vi "XML ( Open ).vi"(8 "error in (no error)":errorcluster, 10 "XML document":path caption="path to XML document", 11 "XML in":refnum<class "XML.lvclass">) -> (0 "error out":errorcluster, 3 "XML out":refnum<class "XML.lvclass">)   [LabVIEW 2018, in "XML.lvlib" / "XML.lvclass"]
uses:
  XML.lvclass
  XML.lvclass/XML.ctl
  <vilib>/xml/Load XML File.vi
  <vilib>/xml/NI_XML.lvlib
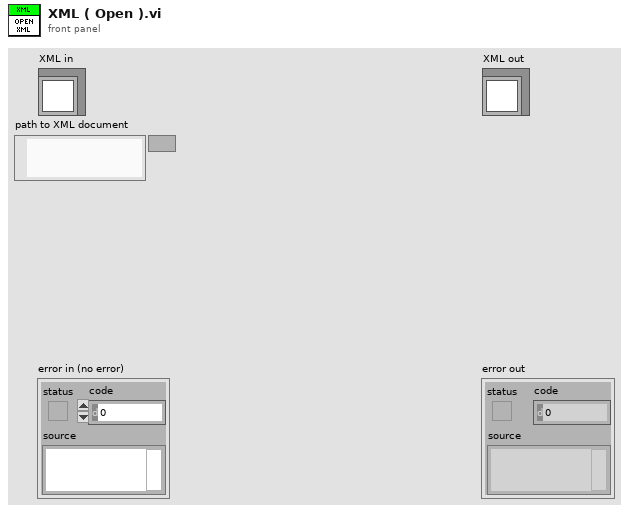
[diagram p1: front panel]
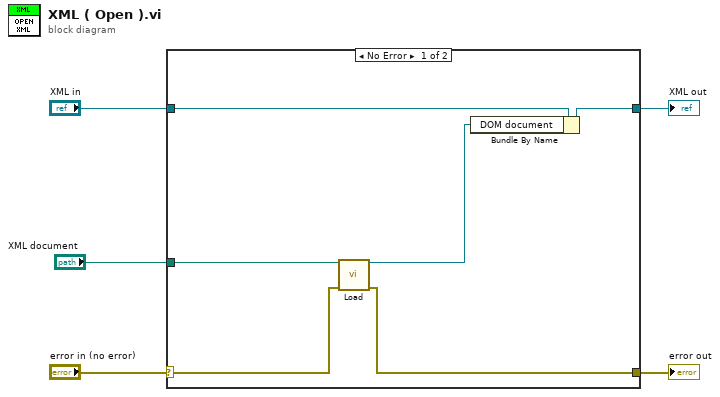
[diagram p0: block diagram]
diagram:
  n1 = case shown="No Error" "error in (no error)" {
    selector: "error in (no error)" -> [w10 w13]
    tunnel: [w9 w13] -> w4
    tunnel: [w7 w12] -> w2
    tunnel: "XML in" -> [w11 w12]
    tunnel: "XML document" -> [w8 _]
    frame No Error {
      n2 = call-poly <vilib>:"Load.vi"("path to XML document"=w8, "error in (no error)"=w10) -> ("DOM document out"=w6:refnum<k20>, "error out"=w9:errorcluster)  [unwired: 11 in, 1 out]
      n3 = Bundle By Name(cluster=w11, "DOM document"=w6) -> (w7:refnum<class "XML.lvclass">)
    }
    frame Error {
    }
  }
  "error out" <- w4
  "XML out" <- w2
